vi "TapeTestProgram.vi"() -> ()   [LabVIEW 2011]
uses:
  TapeDrive/Direction_TypDef.ctl
  TapeDrive/settings_TypDef.ctl
  shared/numericVariable_TypeDef.ctl
  shared/OnOffTypeDef.ctl
  TapeDrive/TapeDrive.lvclass
panel:
  in  "Settings":T1
  in  "stop":bool
  out "Settings":T1
  in  "max velocity":dbl format="%.4g"
  in  "RedRatio":dbl=1.0
  in  "Step":bool
  out "Reduction Ratio":dbl format="%.6g"
  out "max velocity read":dbl format="%.4g"
  in  "direction 2":T4
  out "error out":errorcluster
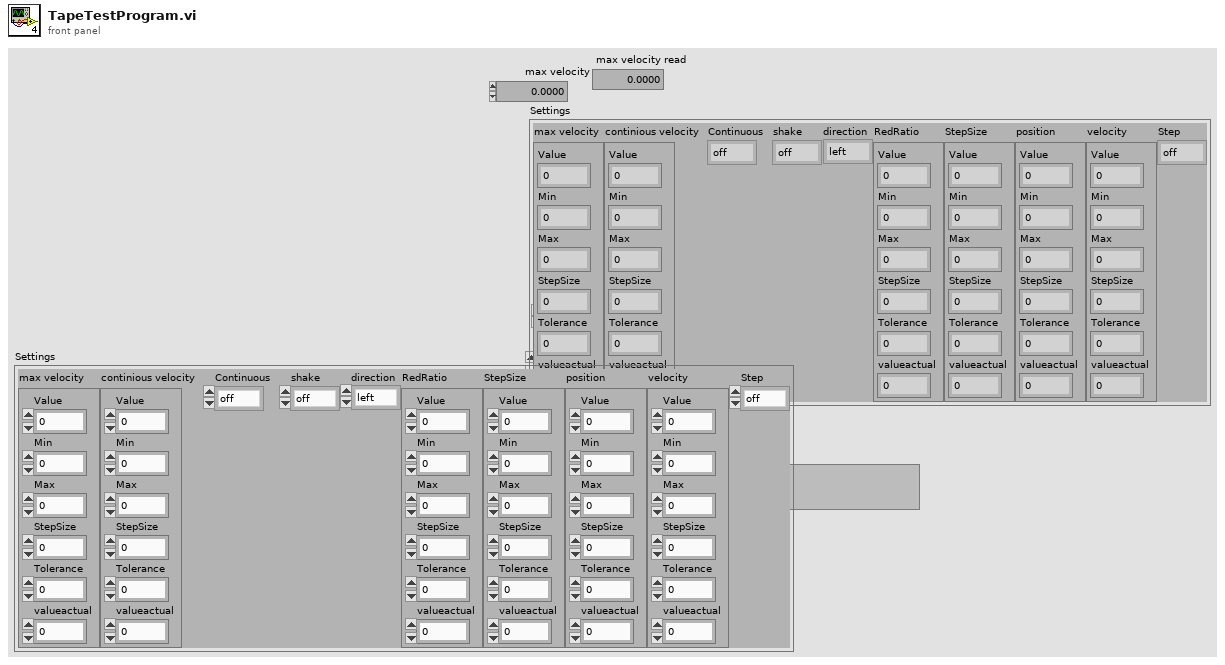
[diagram p1: front panel]
types:
  T1 = typedef "TapeDrive.lvclass/settings_TypDef.ctl" = cluster{"max velocity":T2, "continious velocity":T2, "Continuous":T3, "shake":T3, "direction":T4, "RedRatio":T2, "StepSize":T2, "position":T2, "velocity":T2, "Step":T3}
  T2 = typedef "numericVariable_TypeDef.ctl" = cluster{"Value":dbl, "Min":dbl, "Max":dbl, "StepSize":dbl, "Tolerance":dbl, "valueactual":dbl}
  T3 = typedef "OnOffTypeDef.ctl" = enum16{"off", "on"}
  T4 = typedef "Direction_TypDef.ctl" = enum16{"left", "right"}
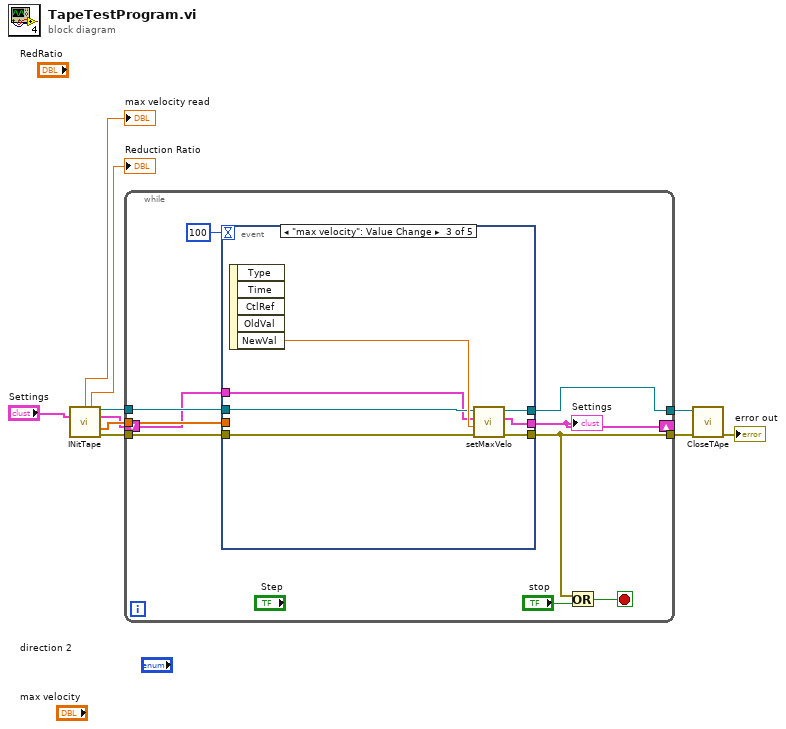
[diagram p0: block diagram]
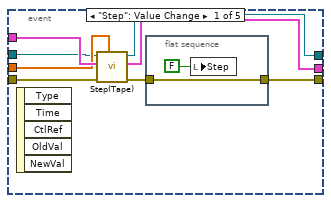
[diagram p2: hidden frame]
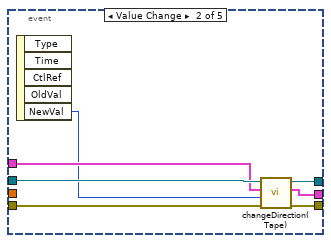
[diagram p3: hidden frame]
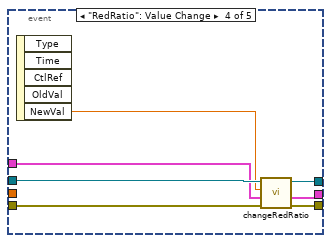
[diagram p4: hidden frame]
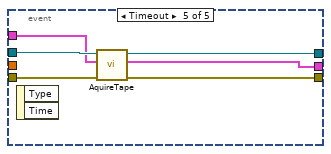
[diagram p5: hidden frame]
diagram:
  n1 = call "INitTape.vi"("Settings in"="Settings") -> ("Velocity (units/s) out"=→"max velocity read":dbl, "Reduction Ratio"=→"Reduction Ratio":dbl, "VISA Refnum out"=w10:refnum<visa-resource-name>, "Settings out"=w2:T1, "downramp array"=w3:dbl[], "error out"=w8:errorcluster)  [unwired: 9 in]
  n2 = while {
    tunnel: w10 -> [w20]
    tunnel: [w19] -> w9
    tunnel: [w16] -> w6
    tunnel: w8 -> [w18]
    tunnel: w3 -> [w14]
    shift-right: [w11] -> _
    shift-left: w2 -> [w12]
    stop <- w13 stop-if-true
    n3 = event shown="[2] \"max velocity\": Value Change" {
      selector: _ -> [_ _ _ _ _]
      dyn-events: _ -> [_ _ _ _ _]
      timeout: 100 -> [_ _ _ _ _]
      tunnel: w20 -> [w23 w35 w40 w51 w57]
      tunnel: [w22 w36 w42 w48 w56] -> w19
      tunnel: w18 -> [w21 w34 w43 w49 w54]
      tunnel: [w25 w37 w41 w47 w55] -> w16
      tunnel: w14 -> [w24 _ _ _ _]
      tunnel: w12 -> [w28 w32 w39 w46 w53]
      tunnel: [w27 w33 w38 w45 w52] -> w11
      event "Step": Value Change {
        n4 = event-data() -> ()  [unwired: 1 in, 5 out]
        n5 = call "Step(Tape).vi"("downramp array"=w24, "error in (no error)"=w21, "Settings"=w28, "VISA resource name"=w23) -> ("error out"=w26:errorcluster, "Settings"=w27:T1, "VISA resource name out"=w22:refnum<visa-resource-name>)  [unwired: 3 in, 2 out]
        n6 = flat-sequence {
          tunnel: w26 -> [w29]
          tunnel: [w29] -> w25
          frame #0 {
            n7 = local write "Step"(FALSE ("Step")) -> ()
          }
        }
      }
      event Value Change {
        n8 = event-data() -> ("NewVal"=w31:T4)  [unwired: 1 in, 4 out]
        n9 = call "changeDirection(Tape).vi"("error in (no error)"=w34, "direction 2"=w31, "Settings"=w32, "VISA Refnum in"=w35) -> ("error out"=w37:errorcluster, "Settings"=w33:T1, "VISA Refnum out"=w36:refnum<visa-resource-name>)  [unwired: 4 in, 1 out]
      }
      event "max velocity": Value Change {
        n10 = event-data() -> ("NewVal"=w44:dbl)  [unwired: 1 in, 4 out]
        n11 = call "setMaxVelo.vi"("error in (no error)"=w43, "NewVal"=w44, "Settings"=w39, "VISA Refnum in"=w40) -> ("error out"=w41:errorcluster, "Settings"=w38:T1, "VISA Refnum out"=w42:refnum<visa-resource-name>)  [unwired: 4 in, 1 out]
      }
      event "RedRatio": Value Change {
        n12 = event-data() -> ("NewVal"=w50:dbl)  [unwired: 1 in, 4 out]
        n13 = call "changeRedRatio.vi"("error in (no error)"=w49, "Settings"=w46, "NewVal"=w50, "VISA Refnum in"=w51) -> ("error out"=w47:errorcluster, "Settings"=w45:T1, "VISA Refnum out"=w48:refnum<visa-resource-name>)  [unwired: 3 in, 2 out]
      }
      event Timeout {
        n14 = event-data() -> ()  [unwired: 1 in, 2 out]
        n15 = call "AquireTape.vi"("error in (no error)"=w54, "Settings"=w53, "VISA Refnum in"=w57) -> ("error out"=w55:errorcluster, "Settings"=w52:T1, "VISA Refnum out"=w56:refnum<visa-resource-name>)  [unwired: 3 in, 3 out]
      }
    }
    "Settings" <- w11
    n16 = Or(x=w16, y="stop") -> (x .or. y?=w13:bool)
  }
  n17 = call "CloseTApe.vi"("error in (no error)"=w6, "VISA Refnum in"=w9) -> ("error out"=→"error out":errorcluster)  [unwired: 9 in]
